vi "nt mode FGV.vi"(7 "Command":T1(ring), 8 "error in (no error)":errorcluster, 10 "Cluster":cluster{"Speed":dbl[], "Torque":dbl[]} {"Torque" format="%_6g"; "Speed" format="%_6g"}, 11 "File Path":path) -> (0 "error out":errorcluster, 2 "Cluster 2":cluster{"Speed":dbl[], "Torque":dbl[]} {"Torque" format="%_6g"; "Speed" format="%_6g"})   [LabVIEW 2018]
doc: "This Subvi usde for CSV Initialize ,Read, Write and close.\nIntilise case; we check File avaliblity in not found create csv file\nRead Case ; Read data from csv file"
uses:
  <vilib>/Utility/file.llb/Write Delimited Spreadsheet (string).vi
  <vilib>/Utility/file.llb/Read Delimited Spreadsheet (string).vi
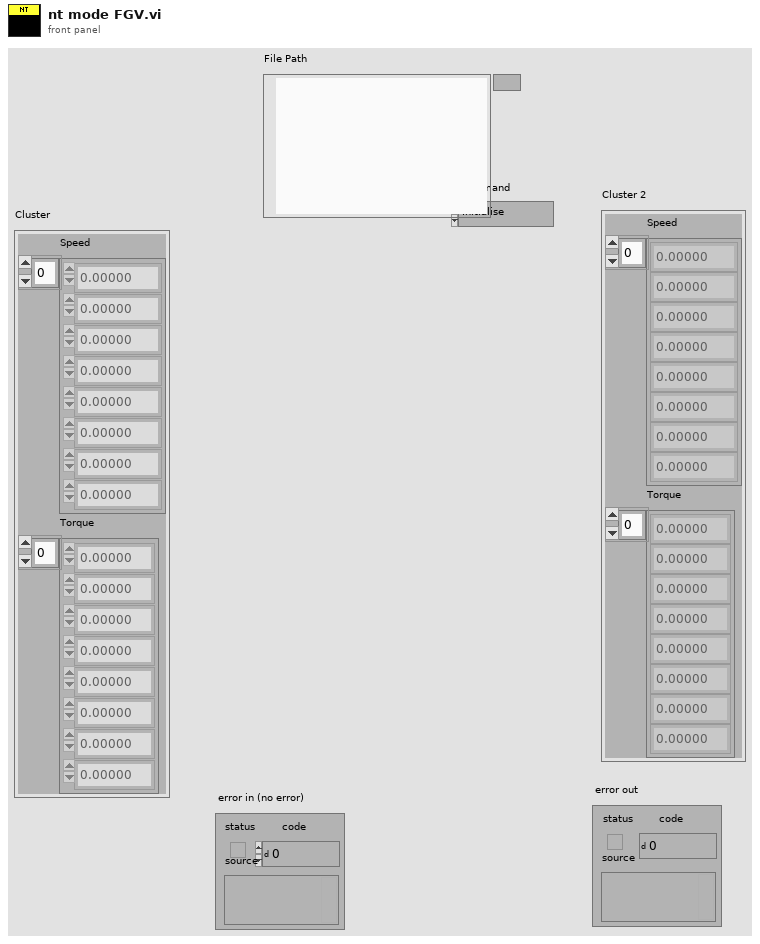
[diagram p1: front panel]
types:
  T1 = enum16{"Initialise", "Read Data", "Write Data", "Close"}
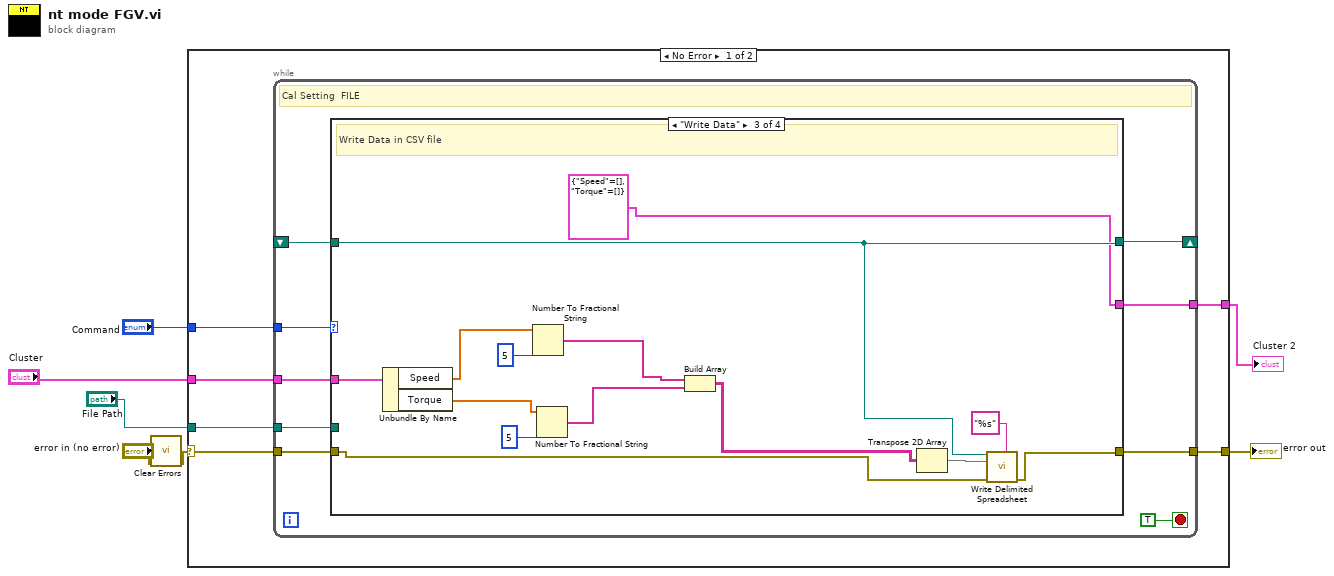
[diagram p0: block diagram]
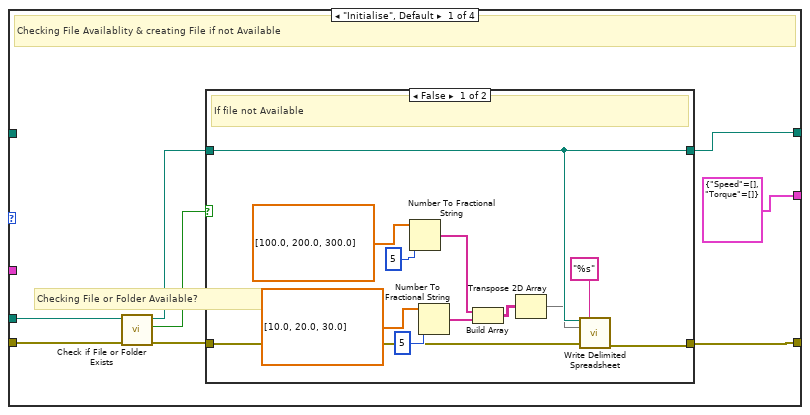
[diagram p2: hidden frame]
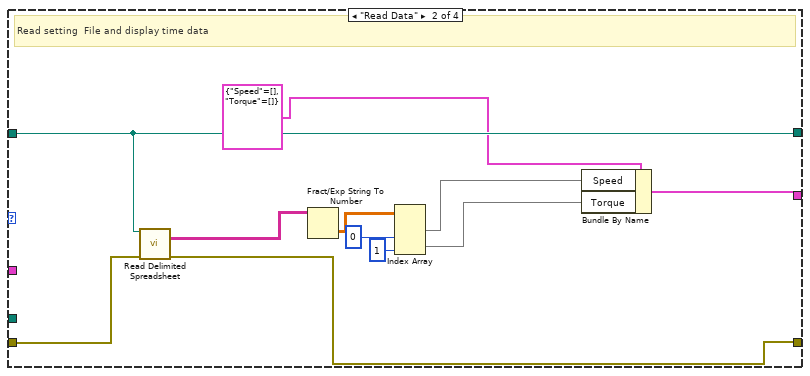
[diagram p4: hidden frame]
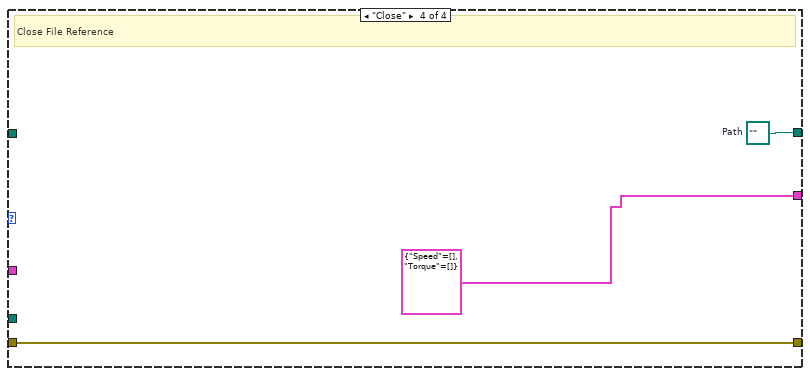
[diagram p5: hidden frame]
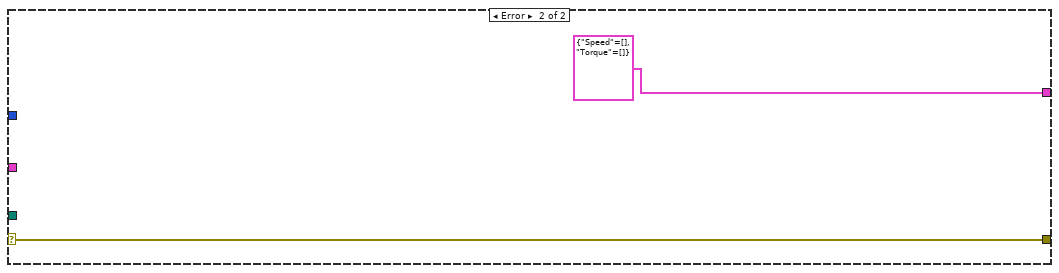
[diagram p6: hidden frame]
diagram:
  n1 = call <vilib>:"Clear Errors.vi"("error in (no error)"="error in (no error)") -> ("error out"=w4:errorcluster)  [unwired: 5 in, 1 out]
  n2 = case shown="No Error" w4 {
    selector: w4 -> [w12 w74]
    tunnel: [w11 w74] -> w6
    tunnel: "Command" -> [w13 _]
    tunnel: "File Path" -> [w10 _]
    tunnel: "Cluster" -> [w9 _]
    tunnel: [w8 cluster{"Speed":dbl[], "Torque":dbl[]} {"Speed"=[], "Torque"=[]} ("Cluster")] -> w2
    frame No Error {
      n3 = while {
        shift-right: [w17] -> _
        shift-left: _ -> [w16]
        tunnel: w13 -> [w21]
        tunnel: w12 -> [w20]
        tunnel: [w19] -> w11
        tunnel: w10 -> [w18]
        tunnel: w9 -> [w15]
        tunnel: [w14] -> w8
        stop <- TRUE stop-if-true
        # "Cal Setting  FILE"
        n4 = case shown="\"Write Data\"" w21 {
          tunnel: w20 -> [w30 w52 w65 w72]
          tunnel: [w24 w51 w64 w72] -> w19
          tunnel: w18 -> [w29 _ _ _]
          tunnel: [w27 w53 w63 w71] -> w17
          tunnel: w16 -> [_ w53 w63 _]
          tunnel: w15 -> [_ _ w60 _]
          tunnel: [cluster{"Speed":dbl[], "Torque":dbl[]} {"Speed"=[], "Torque"=[]} ("Cluster") w54 cluster{"Speed":dbl[], "Torque":dbl[]} {"Speed"=[], "Torque"=[]} ("Cluster") cluster{"Speed":dbl[], "Torque":dbl[]} {"Speed"=[], "Torque"=[]} ("Cluster")] -> w14
          frame "Initialise", Default {
            # "Checking File or Folder Available?"
            # "Checking File Availablity & creating File if not Available"
            n5 = call <vilib>:"Check if File or Folder Exists.vi"("error in (no error)"=w30, "path"=w29) -> ("error out"=w25:errorcluster, "file or folder exists?"=w28:bool, "dup path"=w26:path)  [unwired: 7 in]
            n6 = case shown="False" w28 {
              tunnel: [w38 w44] -> w27
              tunnel: w26 -> [w38 w44]
              tunnel: w25 -> [w35 w43]
              tunnel: [w34 w43] -> w24
              frame False {
                # "If file not Available"
                n7 = Number To Fractional String(number=dbl[] [100.0, 200.0, 300.0], precision (6)=i16 5) -> (F-format string=w31:string[])  [unwired: 2 in]
                n8 = Number To Fractional String(number=dbl[] [10.0, 20.0, 30.0], precision (6)=i16 5) -> (F-format string=w41:string[])  [unwired: 2 in]
                n9 = Build Array(w31, w41) -> (w42:string[][])
                n10 = Transpose 2D Array(2D array=w42) -> (transposed array=w37:string[][])
                n11 = call-poly <vilib>:"Write Delimited Spreadsheet.vi"("file path (dialog if empty)"=w38, "format (%s)"="%s", "2D data"=w37, "error in (no error)"=w35) -> ("error out"=w34:errorcluster)  [unwired: 10 in, 1 out]
              }
              frame True {
                # "If File available"
              }
            }
          }
          frame "Read Data" {
            # "Read setting  File and display time data"
            n12 = call-poly <vilib>:"Read Delimited Spreadsheet.vi"("file path (dialog if empty)"=w53, "error in (no error)"=w52) -> ("all rows"=w50:string[][], "error out"=w51:errorcluster)  [unwired: 8 in, 4 out]
            n13 = Fract/Exp String To Number(string=w50) -> (number=w49:dbl[][])  [unwired: 3 in, 1 out]
            n14 = Index Array(array=w49, index (col) #1=0 ("disabled index (col)"), index (col) #2=1 ("index (col)")) -> (element #1=w47:dbl[], element #2=w46:dbl[])  [unwired: 2 in]
            n15 = Bundle By Name(cluster=cluster{"Speed":dbl[], "Torque":dbl[]} {"Speed"=[], "Torque"=[]} ("Cluster"), "Speed"=w47, "Torque"=w46) -> (w54:cluster{"Speed":dbl[], "Torque":dbl[]})
          }
          frame "Write Data" {
            # "Write Data in CSV file"
            n16 = Unbundle By Name(w60) -> ("Speed"=w57:dbl[], "Torque"=w56:dbl[])
            n17 = Number To Fractional String(number=w57, precision (6)=i16 5) -> (F-format string=w58:string[])  [unwired: 2 in]
            n18 = Number To Fractional String(number=w56, precision (6)=i16 5) -> (F-format string=w69:string[])  [unwired: 2 in]
            n19 = Build Array(w58, w69) -> (w62:string[][])
            n20 = Transpose 2D Array(2D array=w62) -> (transposed array=w67:string[][])
            n21 = call-poly <vilib>:"Write Delimited Spreadsheet.vi"("file path (dialog if empty)"=w63, "format (%s)"="%s", "2D data"=w67, "error in (no error)"=w65) -> ("error out"=w64:errorcluster)  [unwired: 10 in, 1 out]
          }
          frame "Close" {
            w71 = path ""  # Path
            # "Close File Reference"
          }
        }
      }
    }
    frame Error {
    }
  }
  "error out" <- w6
  "Cluster 2" <- w2
